vi "Main.vi"(11 "Module Admin":refnum<class "Delacor_lib_QMH_Module Admin.lvclass">) -> ()   [LabVIEW 2024, in "Acquisition.lvlib"]
doc: "This template is based off of the Queued Message Handler design pattern and the Queued Message Handler project template that ships with LabVIEW.\n\nThe main difference is that the queue is private to this module and communication between modules is performed via Broadcast and Request events.\n\nRequest events are wrapped in public API methods and are handled in the Event Handling Loop (EHL) of this VI. Any module can register for Broadcast events sent by this module. The EHL generates messages based on user interface actions.\n\nThe Message Handling Loop (MHL) processes messages generated by the EHL, or by other messages. The messages are string values, so new messages can be added easily to the Message Cases case structure in the MHL. Each message cluster can also provide an optional value for Message Data, which is a variant that can be converted to whatever message-specific data is required.\n_____\nBased on DQMH Project Template 4.0.0.47.\n_____\nBased on DQMH Project Template 7.0.1.1316."
uses:
  Acquisition.lvlib
  <vilib>/Delacor/Delacor QMH/Libraries/Module Admin_class/Delacor_lib_QMH_Module Admin.lvclass
  Module Data--cluster.ctl
  CML Shared/Signal Type--enum.ctl
  CML Shared/Calibration Values--cluster.ctl
  Stop Argument--cluster.ctl
  <vilib>/Delacor/Delacor QMH/Libraries/Message Queue_class/Delacor_lib_QMH_Message Queue.lvclass/Delacor_lib_QMH_Message Queue.ctl
  <vilib>/Delacor/Delacor QMH/Libraries/Module Admin_class/Delacor_lib_QMH_Module Admin.lvclass/Delacor_lib_QMH_Module Admin.ctl
  Start Acquiring Argument--cluster.ctl
  Start Acquiring (Reply Payload)--cluster.ctl
  Stop Acquiring Argument--cluster.ctl
  Settings Editor/Update Application Settings (Reply Payload)--cluster.ctl
  Settings Editor/Settings--cluster.ctl
  <vilib>/Utility/miscctls.llb/LVPointTypeDef.ctl
  <vilib>/Delacor/Delacor QMH/Libraries/Message Queue_class/Delacor_lib_QMH_Enqueue Message (Single).vi
  <vilib>/Delacor/Delacor QMH/Libraries/Module Admin_class/Delacor_lib_QMH_Get External Launch.vi
  <vilib>/Delacor/Delacor QMH/Libraries/Message Queue_class/Delacor_lib_QMH_Message Queue.lvclass
  CML Shared/CML Shared.lvlib
  Settings Editor/Settings Editor.lvlib
  Logger/Logger.lvlib
panel:
  out "Settings":T1
  out "Graph Data":waveform(dbl)[](array[waveform])
  out "error out":errorcluster
  # "This is a headless module. Show its panel to confirm that the Settings are updated correctly and other debugging tasks. Use the Settings Editor to change the settings for this module."
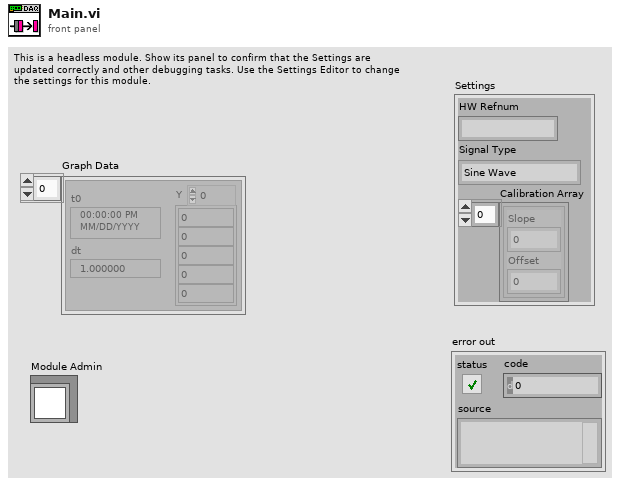
[diagram p1: front panel]
types:
  T1 = typedef "Acquisition.lvlib/Module Data--cluster.ctl" = cluster{"HW Refnum":string, "Signal Type":T2, "Calibration Array":T3[]}
  T2 = typedef "CML Shared.lvlib/Signal Type--enum.ctl" = enum16{"Sine Wave", "Square with Noise"}
  T3 = typedef "CML Shared.lvlib/Calibration Values--cluster.ctl" = cluster{"Slope":dbl, "Offset":dbl}
  T4 = typedef "Settings Editor.lvlib/Broadcast Events--cluster.ctl" = cluster{"Module Did Init":refnum<user-event>, "Status Updated":refnum<user-event>, "Error Reported":refnum<user-event>, "Module Did Stop":refnum<user-event>, "Update Module Execution Status":refnum<user-event>, "Application Settings Updated":refnum<user-event>}
  T5 = typedef "Acquisition.lvlib/Request Events--cluster.ctl" = cluster{"Stop Module":refnum<user-event>, "Show Panel":refnum<user-event>, "Hide Panel":refnum<user-event>, "Get Module Execution Status":refnum<user-event>, "Show Diagram":refnum<user-event>, "Stop Acquiring":refnum<user-event>, "Wakeup Helper Loop":refnum<user-event>, "Change Settings":refnum<user-event>, "Calibrate DAQ":refnum<user-event>, "Start Acquiring":refnum<user-event>}
  T6 = enum32{"invalid lock state", "Not Locked", "Locked (No Password)", "Password-protected"}
  T7 = typedef "Acquisition.lvlib/Stop Argument--cluster.ctl" = cluster{"Origin":string, "Exit via Stop Module Req?":bool, "Wait for Module to stop?":bool}
  T8 = typedef "Acquisition.lvlib/Start Acquiring Argument--cluster.ctl" = cluster{"Wait Notifier":refnum<notifier>, "wait for reply":bool}
  T9 = typedef "Acquisition.lvlib/Stop Acquiring Argument--cluster.ctl" = cluster{"Boolean":bool}
  T10 = typedef "Settings Editor.lvlib/Update Application Settings (Reply Payload)--cluster.ctl" = cluster{"Settings":T11, "error":errorcluster}
  T11 = typedef "Settings Editor.lvlib/Settings--cluster.ctl" = cluster{"Signal Type":T2, "Calibration Array":T3[], "Log File Base Path":path}
  T12 = typedef "LVPointTypeDef.ctl" = cluster{"Horizontal":i16, "Vertical":i16}
  T13 = enum32{"Invalid", "Standard", "Closed", "Hidden", "Minimized", "Maximized"}
  T14 = typedef "Acquisition.lvlib/Start Acquiring (Reply Payload)--cluster.ctl" = cluster{"HW ID":string, "error":errorcluster}
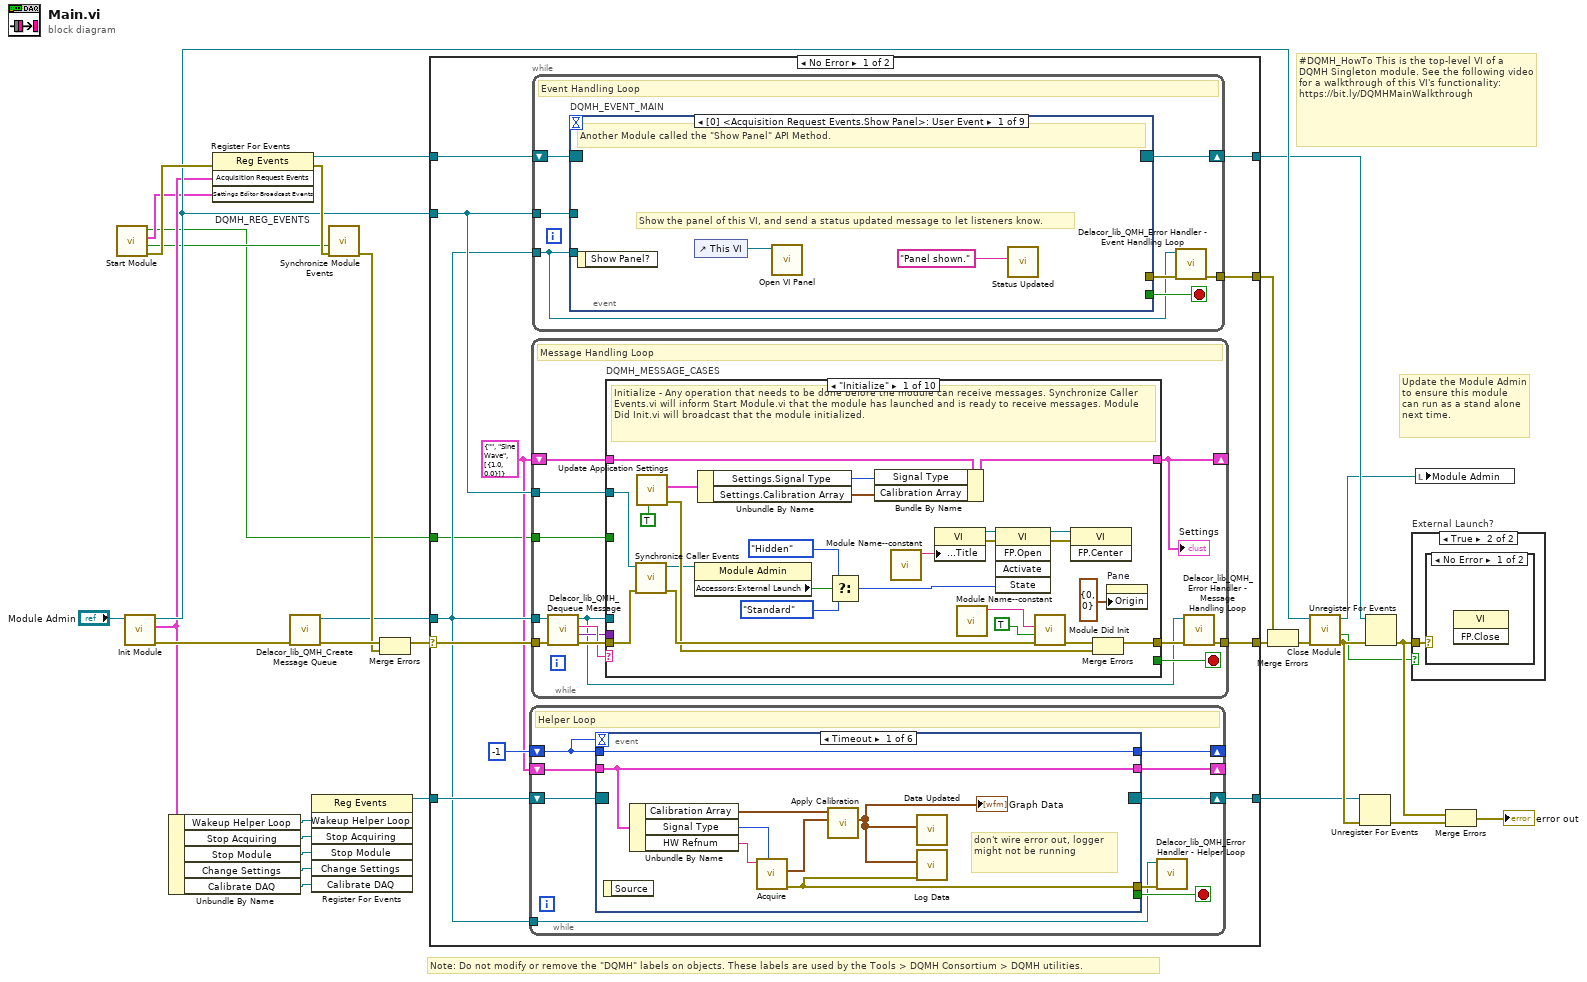
[diagram p0: block diagram]
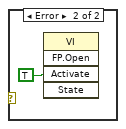
[diagram p3: hidden frame]
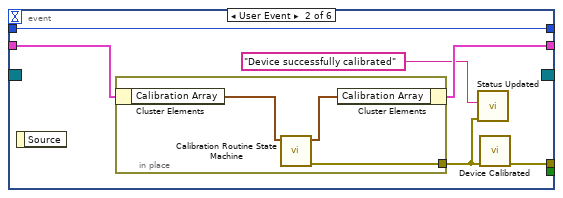
[diagram p4: hidden frame]
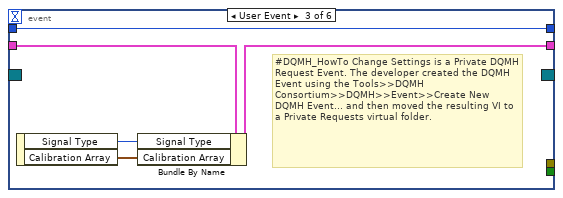
[diagram p5: hidden frame]
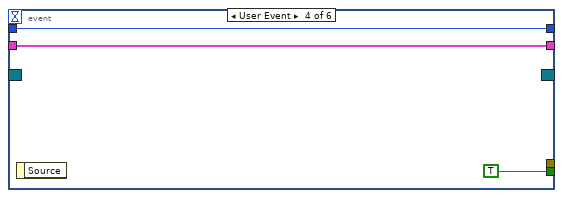
[diagram p6: hidden frame]
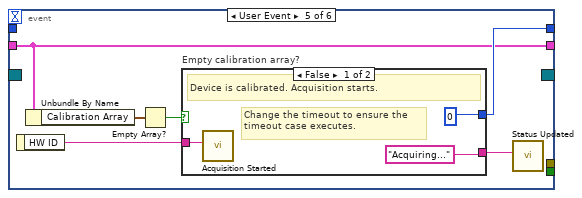
[diagram p7: hidden frame]
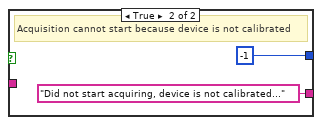
[diagram p8: hidden frame]
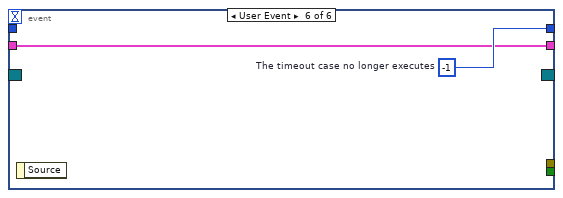
[diagram p9: hidden frame]
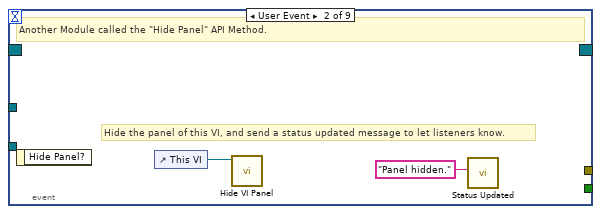
[diagram p10: hidden frame]
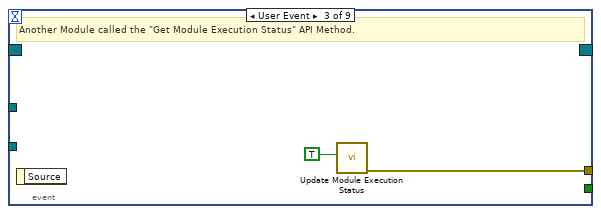
[diagram p11: hidden frame]
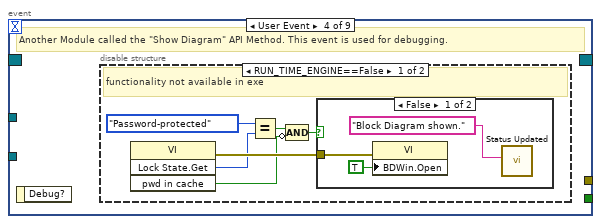
[diagram p12: hidden frame]
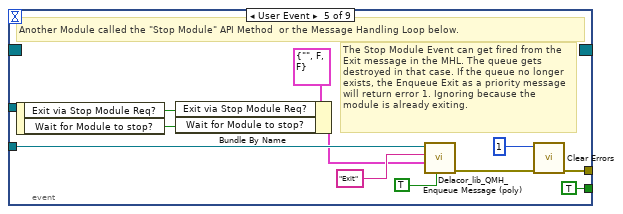
[diagram p15: hidden frame]
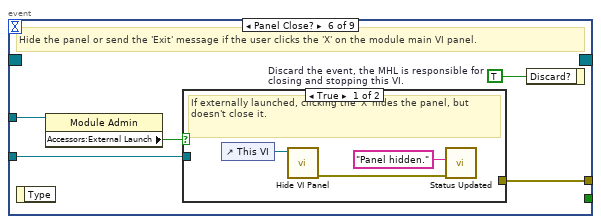
[diagram p16: hidden frame]
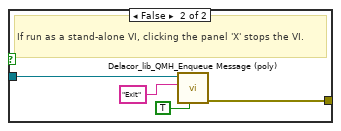
[diagram p17: hidden frame]
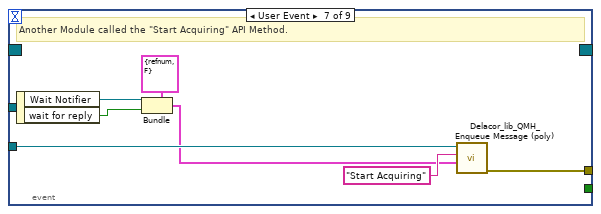
[diagram p18: hidden frame]
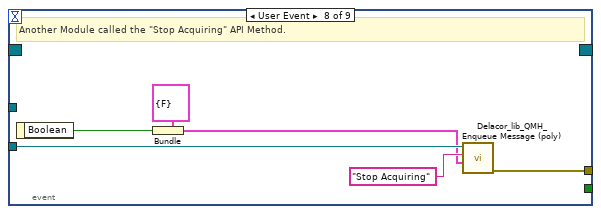
[diagram p19: hidden frame]
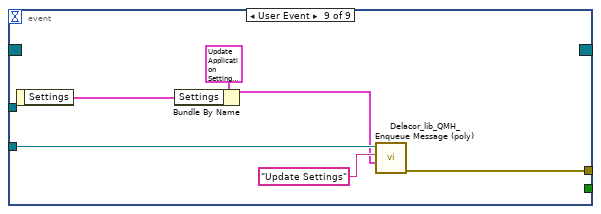
[diagram p20: hidden frame]
diagram:
  # "#DQMH_HowTo This is the top-level VI of a DQMH Singleton module. See the following video for a walkthrough of this VI's functionality: https://bit.ly/DQMHMainWalkthrough"
  # "Note: Do not modify or remove the \"DQMH\" labels on objects. These labels are used by the Tools > DQMH Consortium > DQMH utilities."
  # "Update the Module Admin to ensure this module can run as a stand alone next time."
  n1 = call "Start Module.vi"() -> ("error out"=w24:errorcluster, "Wait for Event Sync?"=w5:bool, "Settings Editor Broadcast Events"=w6:T4, "Module Was Already Running?"=w1:bool)  [unwired: 8 in]
  n2 = call "Init Module.vi"("Singleton Module Admin in"="Module Admin") -> ("error out"=w30:errorcluster, "Acquisition Request Events"=w11:T5, "Singleton Module Admin out"=w18:refnum<class "Delacor_lib_QMH_Module Admin.lvclass">)  [unwired: 8 in]
  n3 = Unbundle By Name(w11) -> ("Wakeup Helper Loop"=w7:refnum<user-event>, "Stop Acquiring"=w10:refnum<user-event>, "Stop Module"=w9:refnum<user-event>, "Change Settings"=w4:refnum<user-event>, "Calibrate DAQ"=w3:refnum<user-event>)
  n4 = register-events "DQMH_REG_EVENTS"(error in=w24, w11, w6) -> (reference out=w16:refnum<event-registration>, error out=w23:errorcluster)  [unwired: 1 in]
  n5 = call <vilib>:"Delacor_lib_QMH_Create Message Queue.vi"("error in"=w30) -> ("error out"=w26:errorcluster, "Message Queue"=w15:refnum<class "Delacor_lib_QMH_Message Queue.lvclass">)  [unwired: 9 in]
  n6 = register-events(w7, w10, w9, w4, w3) -> (reference out=w8:refnum<event-registration>)  [unwired: 2 in, 1 out]
  n7 = call "Synchronize Module Events.vi"("error in"=w23, "Wait for Event Sync?"=w5) -> ("error out"=w22:errorcluster)  [unwired: 9 in]
  n8 = Merge Errors(w26, w22) -> (w25:errorcluster)
  n9 = case shown="No Error" w25 {
    selector: w25 -> [w41 w293]
    tunnel: [w43 w292] -> w31
    tunnel: [w40 w291] -> w17
    tunnel: w16 -> [w39 w291]
    tunnel: w15 -> [w35 w284]
    tunnel: [w42 _] -> w29
    tunnel: w18 -> [w38 w287]
    tunnel: w8 -> [w36 w286]
    tunnel: [w33 w286] -> w2
    tunnel: w1 -> [w32 w285]
    frame No Error {
      w34 = T1 {"HW Refnum"="", "Signal Type"=enum."Sine Wave", "Calibration Array"=[{"Slope"=1.0, "Offset"=0.0}]} ("Data Cluster")
      n10 = while {
        shift-right: [w51] -> _
        shift-left: -1 -> [w50]
        tunnel: w35 -> [w44]
        shift-right: [w47] -> _
        shift-left: w34 -> [w46]
        shift-right: [w45] -> w33
        shift-left: w36 -> [w49]
        stop <- w48 stop-if-true
        # "Helper Loop"
        n11 = event shown="[0] Timeout" {
          selector: w49 -> [_ _ _ _ _ _]
          dyn-events: [_ _ _ _ _ _] -> w45
          timeout: w50 -> [_ _ _ _ _ _]
          tunnel: [w59 w64 w74 w77 w82 w90] -> w51
          tunnel: w50 -> [w59 w64 w74 w77 _ _]
          tunnel: [_ _ _ TRUE _ _] -> w48
          tunnel: [w60 w66 _ _ _ _] -> w52
          tunnel: [w56 w62 w72 w75 w79 w89] -> w47
          tunnel: w46 -> [w56 w63 w73 w75 w79 w89]
          event Timeout {
            # "don't wire error out, logger might not be running"
            n12 = event-data() -> ()  [unwired: 1 in, 1 out]
            n13 = Unbundle By Name(w56) -> ("Calibration Array"=w54:T3[], "Signal Type"=w58:T2, "HW Refnum"=w57:string)
            n14 = call "Acquire.vi"("Signal Type"=w58, "HW ID in"=w57) -> ("error out"=w60:errorcluster, "Graph Data"=w55:waveform(dbl)[])  [unwired: 7 in, 1 out]
            n15 = call "Apply Calibration.vi"("Graph Data"=w55, "Calibration Array"=w54) -> ("Calibrated Data"=w53:waveform(dbl)[])  [unwired: 9 in]
            "Graph Data" <- w53
            n16 = call "Data Updated.vi"("Graph Data"=w53) -> ()  [unwired: 10 in, 1 out]
            n17 = call "Log Data.vi"("error in"=w60, "Waveforms"=w53) -> ()  [unwired: 9 in, 1 out]
          }
          event User Event {
            n18 = event-data() -> ()  [unwired: 1 in, 1 out]
            n19 = in-place {
              in-place-border: [w69] -> w65
              n20 = in-place-cluster #1(w63) -> ("Calibration Array"=w68:T3[])
              n21 = call "Calibration Routine State Machine.vi"("Calibration Array in"=w68) -> ("error out"=w69:errorcluster, "Calibration Array out"=w67:T3[])  [unwired: 9 in]
              n22 = in-place-cluster #1("Calibration Array"=w67) -> (w62:T1)
            }
            n23 = call "Status Updated.vi"("error in"=w65, "Status"="Device successfully calibrated") -> ()  [unwired: 9 in, 1 out]
            n24 = call "Device Calibrated.vi"("error in"=w65) -> ("error out"=w66:errorcluster)  [unwired: 10 in]
          }
          event User Event {
            # "#DQMH_HowTo Change Settings is a Private DQMH Request Event. The developer created the DQMH Event using the Tools>>DQMH Consortium>>DQMH>>Event>>Create New DQMH Event... and then moved the resulting VI to a Private Requests virtual folder."
            n25 = event-data() -> ("Signal Type"=w71:T2, "Calibration Array"=w70:T3[])  [unwired: 1 in]
            n26 = Bundle By Name(cluster=w73, "Signal Type"=w71, "Calibration Array"=w70) -> (w72:T1)
          }
          event User Event {
            n27 = event-data() -> ()  [unwired: 1 in, 1 out]
          }
          event User Event {
            n28 = event-data() -> ("HW ID"=w80:string)  [unwired: 1 in]
            n29 = Unbundle By Name(w79) -> ("Calibration Array"=w78:T3[])
            n30 = Empty Array?(array=w78) -> (empty?=w83:bool)
            n31 = case "Empty calibration array?" shown="False" w83 {
              tunnel: ["Acquiring..." ("Status") "Did not start acquiring, device is not calibrated..." ("Status")] -> w81
              tunnel: [0 -1] -> w82
              tunnel: w80 -> [w86 _]
              frame False {
                # "Change the timeout to ensure the timeout case executes."
                # "Device is calibrated. Acquisition starts."
                n32 = call "Acquisition Started.vi"("HW ID"=w86) -> ()  [unwired: 10 in, 1 out]
              }
              frame True {
                # "Acquisition cannot start because device is not calibrated"
              }
            }
            n33 = call "Status Updated.vi"("Status"=w81) -> ()  [unwired: 10 in, 1 out]
          }
          event User Event {
            w90 = -1  # The timeout case no longer executes
            n34 = event-data() -> ()  [unwired: 1 in, 1 out]
          }
        }
        n35 = call-dynamic "Delacor_lib_QMH_Error Handler - Helper Loop.vi"("error in"=w52, "Message Queue in"=w44) -> ()  [unwired: 8 in, 2 out]
      }
      n36 = while {
        tunnel: w35 -> [w158]
        shift-right: [w162] -> _
        shift-left: w34 -> [w163]
        tunnel: w41 -> [w166]
        tunnel: [w164] -> w43
        tunnel: w38 -> [w156]
        tunnel: w32 -> [w155]
        stop <- w161 stop-if-true
        # "Message Handling Loop"
        n37 = call-dynamic "Delacor_lib_QMH_Dequeue Message.vi"("error in"=w166, "Message Queue in"=w158) -> ("error out"=w165:errorcluster, "Message Data"=w159:variant, "Message"=w160:string, "Message Queue out"=w157:refnum<class "Delacor_lib_QMH_Message Queue.lvclass">)  [unwired: 6 in]
        n38 = case "DQMH_MESSAGE_CASES" shown="\"Initialize\"" w160 {
          selector: w160 -> [_ _ _ _ _ _ _ _ _ w279]
          tunnel: w157 -> [_ _ _ _ _ _ _ w240 w264 _]
          tunnel: w165 -> [w190 w194 w207 w221 w231 w234 w236 w247 w271 w282]
          tunnel: [w187 w194 w205 w219 w229 w233 w236 w243 w265 w283] -> w167
          tunnel: w163 -> [w177 w193 w195 w216 w227 w232 w235 w242 w256 w280]
          tunnel: [w172 w193 w203 w216 w227 w232 w235 w242 w256 w280] -> w162
          tunnel: [_ _ _ _ _ _ _ _ w263 _] -> w161
          tunnel: w159 -> [_ _ w202 w218 w228 _ _ w241 w262 _]
          tunnel: w156 -> [w178 _ _ _ _ _ _ w239 w257 _]
          tunnel: w155 -> [_ _ _ _ _ _ _ _ w254 _]
          frame "Initialize" {
            # "Initialize - Any operation that needs to be done before the module can receive messages. Synchronize Caller Events.vi will inform Start Module.vi that the module has launched and is ready to receive messages. Module Did Init.vi will broadcast that the module initialized."
            n39 = call "Synchronize Caller Events.vi"("error in"=w190, "Singleton Module Admin in"=w178) -> ("error out"=w189:errorcluster, "Singleton Module Admin out"=w174:refnum<class "Delacor_lib_QMH_Module Admin.lvclass">)  [unwired: 8 in]
            n40 = call "Update Application Settings.vi"("wait for reply (T)"=TRUE) -> ("error out"=w186:errorcluster, "Reply Payload"=w171:T10)  [unwired: 8 in, 1 out]
            n41 = property on="Property Node" class="Module Admin"(reference=w174) -> ("Accessors:External Launch"=w182:bool)  [unwired: 1 in, 2 out]
            n42 = Unbundle By Name(w171) -> ("Settings.Signal Type"=w170:T2, "Settings.Calibration Array"=w169:T3[])
            n43 = Select(t=T13."Hidden" ("State"), s=w182, f=T13."Standard" ("State")) -> (s? t:f=w179:T13)
            n44 = Bundle By Name(cluster=w177, "Signal Type"=w170, "Calibration Array"=w169) -> (w172:T1)
            n45 = call "Module Name--constant.vi"() -> ("Module Name"=w185:string)  [unwired: 11 in]
            n46 = property on="Property Node" class="VI"("Front Panel.Title"=w185) -> (reference out=w184:refnum<vi>, error out=w192:errorcluster)  [unwired: 2 in]
            n47 = call "Module Name--constant.vi"() -> ("Module Name"=w175:string)  [unwired: 11 in]
            n48 = invoke on="Invoke Node" class="VI" method="FP.Open"(reference=w184, error in=w192, "State"=w179) -> (reference out=w183:refnum<vi>, error out=w191:errorcluster)  [unwired: 2 in, 3 out]
            n49 = call "Module Did Init.vi"("error in"=w189, "Initialized?"=TRUE, "Origin"=w175) -> ("error out"=w188:errorcluster)  [unwired: 8 in]
            n50 = invoke on="Invoke Node" class="VI" method="FP.Center"(reference=w183, error in=w191) -> ()  [unwired: 1 in, 3 out]
            n51 = Merge Errors(w188, w186) -> (w187:errorcluster)
            n52 = property on="Pane" class="Pane"("Origin"=T12 {"Horizontal"=0, "Vertical"=0}) -> ()  [unwired: 2 in, 2 out]
          }
          frame "---Module Specific---" {
            # "Separator -- The following cases handle messages specific to this Module."
          }
          frame "Start Acquiring" {
            # "Requests Acquisition Module to start acquiring."
            n53 = Variant To Data(error in=w207, type=T8 {"Wait Notifier"=refnum, "wait for reply"=FALSE} ("Start Acquisition Argument"), Variant=w202) -> (data=w200:T8, error out=w204:errorcluster)
            n54 = in-place {
              in-place-border: [w213] -> w206
              in-place-border: w204 -> [w212]
              in-place-border: [w208] -> w196
              n55 = in-place-cluster #2(w195) -> ("HW Refnum"=w209:string)
              n56 = call "Initialize Hardware References.vi"("error in"=w212, "HW Refnum in"=w209) -> ("error out"=w211:errorcluster, "HW Refnum out"=w210:string)  [unwired: 8 in]
              n57 = call "Configure Hardware.vi"("error in"=w211, "HW Refnum in"=w210) -> ("error out"=w213:errorcluster, "HW Refnum out"=w208:string)  [unwired: 8 in]
              n58 = in-place-cluster #2("HW Refnum"=w208) -> (w203:T1)
            }
            n59 = Unbundle By Name(w200) -> ("Wait Notifier"=w199:refnum<notifier>)
            n60 = call "Wakeup Helper Loop.vi"("error in"=w206, "HW ID"=w196) -> ("error out"=w205:errorcluster)  [unwired: 9 in]
            n61 = Bundle By Name(cluster=T14 {"HW ID"="", "error"={"status"=FALSE, "code"=0, "source"=""}} ("Start Acquisition (Reply Payload)"), "HW ID"=w196, "error"=w206) -> (w198:T14)
            n62 = Send Notification(notification=w198, notifier=w199) -> ()  [unwired: 1 in, 2 out]
          }
          frame "Stop Acquiring" {
            # "Requests the Acquisition Module to stop acquiring"
            n63 = Variant To Data(error in=w221, type=T9 {"Boolean"=FALSE} ("Stop Acquiring Argument"), Variant=w218) -> (error out=w220:errorcluster)  [unwired: 1 out]
            n64 = Unbundle By Name(w216) -> ("HW Refnum"=w215:string)
            n65 = call "Stop Acquisition.vi"("error in"=w220, "HW Refnum"=w215) -> ("error out"=w219:errorcluster)  [unwired: 9 in]
            n66 = call "Acquisition Stopped.vi"("error in"=w219) -> ()  [unwired: 10 in, 1 out]
            n67 = call "Status Updated.vi"("error in"=w219, "Status"="Acquisition Stopped") -> ()  [unwired: 9 in, 1 out]
          }
          frame "Update Settings" {
            # "Send the Change Settings event to the helper loop."
            # "The Settings Editor broadcasted that the settings have changed."
            n68 = Variant To Data(error in=w231, type=T10 {"Settings"={"Signal Type"=enum."Sine Wave", "Calibration Array"=[], "Log File Base Path"=path ""}, "error"={"status"=FALSE, "code"=0, "source"=""}} ("Settings Updated Argument"), Variant=w228) -> (data=w225:T10, error out=w230:errorcluster)
            n69 = Unbundle By Name(w225) -> ("Settings.Signal Type"=w224:T2, "Settings.Calibration Array"=w222:T3[])
            n70 = call "Change Settings.vi"("error in"=w230, "Calibration Array"=w222, "Signal Type"=w224) -> ("error out"=w229:errorcluster)  [unwired: 8 in]
            n71 = call "Status Updated.vi"("error in"=w229, "Status"="Settings Updated") -> ()  [unwired: 9 in, 1 out]
          }
          frame "---Copy This Frame---" {
            # "Duplicate this frame when creating new messages.  Change this comment in the duplicated frame to describe this message."
            n72 = Merge Errors(w234) -> (w233:errorcluster)
          }
          frame "---Exit and Error Handling---" {
            # "Separator - The following cases handle errors and exit messages."
          }
          frame "Error" {
            # "Error - Check the error message data and respond accordingly. This message is sent by the \"Error Handler\" VIs at the end of each loop in this application."
            n73 = property on="Property Node" class="Module Admin"(reference=w239) -> ("Accessors:External Launch"=w238:bool)  [unwired: 1 in, 2 out]
            n74 = Variant To Data(error in=w247, type=errorcluster {"status"=FALSE, "code"=0, "source"=""} ("error constant"), Variant=w241) -> (data=w237:errorcluster, error out=w245:errorcluster)
            n75 = local write "error out"(w237) -> ()
            n76 = call "Error Reported.vi"("Error"=w237) -> ()  [unwired: 10 in, 1 out]
            n77 = case shown="False" w238 {
              tunnel: [w252 _] -> w244
              tunnel: w240 -> [w250 _]
              tunnel: w237 -> [w251 _]
              frame False {
                n78 = disable-structure shown="Default" {
                  disable-tunnel: w251 -> [w253 _]
                  frame condition #0 (active) {
                    # "If the module is running standalone, then pop up an error dialog and call the \"Exit\" message."
                    n79 = call <vilib>:"Simple Error Handler.vi"("error in (no error)"=w253) -> ()  [unwired: 4 in, 5 out]
                  }
                  frame condition #1 {
                    # "To prevent the Simple Error Handler VI from being loaded (e.g. when deploying to a Real-Time target), add the Conditional Disable Symbol \"DQMH_Disable_SEH\" to your project and set it to TRUE."
                  }
                }
                n80 = call-poly <vilib>:"Delacor_lib_QMH_Enqueue Message (poly).vi"("Priority Message? (F)"=TRUE, "Message"="Exit", "Message Queue in"=w250) -> ("error out"=w252:errorcluster)  [unwired: 7 in, 1 out]
              }
              frame True {
                # "If the module was launched externally, calling the Error Reported broadcast VI is the only action performed by the \"Error\" message. The module's caller can then process the error appropriately."
              }
            }
            n81 = Merge Errors(w245, w244) -> (w243:errorcluster)
          }
          frame "Exit" {
            w263 = TRUE  # Stop the VI
            # "Release the message queue reference"
            # "Exit - Exit the application."
            n82 = Variant To Data(error in=w271, type=T7 {"Origin"="", "Exit via Stop Module Req?"=FALSE, "Wait for Module to stop?"=FALSE} ("Stop Argument"), Variant=w262) -> (data=w259:T7, error out=w268:errorcluster)
            n83 = call <vilib>:"Clear Errors.vi"("error in (no error)"=w268, "specific error code to clear (0: all)"=91 ("91: not all Exit messages will have an argument")) -> ("error out"=w270:errorcluster)  [unwired: 4 in, 1 out]
            n84 = Unbundle By Name(w256) -> ("HW Refnum"=w255:string)
            n85 = control-ref of="This VI"() -> (w258:refnum<vi>)
            n86 = call "Handle Exit.vi"("Stop Argument"=w259, "Admin in"=w257, "VI reference"=w258) -> ("error out"=w267:errorcluster)  [unwired: 7 in, 1 out]
            n87 = call "Close Hardware References.vi"("HW Refnum in"=w255) -> ("error out"=w266:errorcluster)  [unwired: 9 in, 1 out]
            n88 = call-dynamic "Delacor_lib_QMH_Release Message Queue.vi"("error in"=w270, "Message Queue"=w264) -> ("error out"=w269:errorcluster)  [unwired: 9 in]
            n89 = case "Settings Editor was\nalready running?" shown="False" w254 {
              frame False {
                n90 = call "Module Name--constant.vi"() -> ("Module Name"=w273:string)  [unwired: 11 in]
                n91 = call "Stop Module.vi"("Wait for Module to Stop? (F)"=TRUE, "Origin"=w273) -> ()  [unwired: 9 in, 1 out]
              }
              frame True {
                # "Another Module stops the Settings Editor"
              }
            }
            n92 = Merge Errors(w269, w267, w266) -> (w265:errorcluster)
            n93 = call "Error Reported.vi"("Error"=w265) -> ()  [unwired: 10 in, 1 out]
          }
          frame Default {
            # "'Default' case only runs if there is a message that isn't defined in any of the other cases.  Output a programming error."
            n94 = call "Module Name--constant.vi"() -> ("Module Name"=w278:string)  [unwired: 11 in]
            n95 = Format Into String(format string="The invalid message string \"%s\" was received in the Message Handling Loop for module \"%s\".", w279, w278) -> (resulting string=w276:string)  [unwired: 2 in, 1 out]
            n96 = call <vilib>:"Error Cluster From Error Code.vi"("show call chain? (False)"=TRUE, "error message (\"\")"=w276, "error code (0)"=1) -> ("error out"=w281:errorcluster)  [unwired: 6 in]
            n97 = Merge Errors(w282, w281) -> (w283:errorcluster)
          }
        }
        "Settings" <- w162
        n98 = call-dynamic "Delacor_lib_QMH_Error Handler - Message Handling Loop.vi"("error in"=w167, "Message Queue in"=w157) -> ("dup error in"=w164:errorcluster)  [unwired: 8 in, 1 out]
      }
      n99 = while {
        tunnel: w35 -> [w91]
        shift-right: [w94] -> w40
        shift-left: w39 -> [w95]
        tunnel: [w96] -> w42
        tunnel: w38 -> [w92]
        stop <- w93 stop-if-true
        # "Event Handling Loop"
        n100 = event "DQMH_EVENT_MAIN" shown="[0] <Acquisition Request Events.Show Panel>: User Event" {
          selector: w95 -> [_ _ _ _ _ _ _ _ _]
          dyn-events: [_ _ _ _ _ _ _ _ _] -> w94
          timeout: _ -> [_ _ _ _ _ _ _ _ _]
          tunnel: [_ _ _ _ TRUE ("Discard?") _ _ _ _] -> w93
          tunnel: w91 -> [_ _ _ _ w119 w126 w141 w147 w152]
          tunnel: [_ _ w103 _ w122 w128 w142 w148 w154] -> w97
          tunnel: w92 -> [_ _ _ _ _ w125 _ _ _]
          event User Event {
            # "Show the panel of this VI, and send a status updated message to let listeners know."
            # "Another Module called the \"Show Panel\" API Method."
            n101 = event-data() -> ()  [unwired: 1 in, 1 out]
            n102 = control-ref of="This VI"() -> (w99:refnum<vi>)
            n103 = call "Open VI Panel.vi"("VI"=w99) -> ()  [unwired: 10 in, 1 out]
            n104 = call "Status Updated.vi"("Status"="Panel shown." ("format string")) -> ()  [unwired: 10 in, 1 out]
          }
          event User Event {
            # "Hide the panel of this VI, and send a status updated message to let listeners know."
            # "Another Module called the \"Hide Panel\" API Method."
            n105 = event-data() -> ()  [unwired: 1 in, 1 out]
            n106 = control-ref of="This VI"() -> (w101:refnum<vi>)
            n107 = call "Hide VI Panel.vi"("VI"=w101) -> ()  [unwired: 10 in, 1 out]
            n108 = call "Status Updated.vi"("Status"="Panel hidden." ("format string")) -> ()  [unwired: 10 in, 1 out]
          }
          event User Event {
            # "Another Module called the \"Get Module Execution Status\" API Method."
            n109 = event-data() -> ()  [unwired: 1 in, 1 out]
            n110 = call "Update Module Execution Status.vi"("Running?"=TRUE) -> ("error out"=w103:errorcluster)  [unwired: 10 in]
          }
          event User Event {
            # "Another Module called the \"Show Diagram\" API Method. This event is used for debugging."
            n111 = event-data() -> ()  [unwired: 1 in, 1 out]
            n112 = disable-structure shown="RUN_TIME_ENGINE==False" {
              frame condition #0 (active) {
                # "functionality not available in exe"
                n113 = invoke on="Invoke Node" class="VI" method="Lock State.Get"() -> (error out=w109:errorcluster, "Get Lock State"=w108:T6, "pwd in cache"=w105:bool)  [unwired: 4 in, 1 out]
                n114 = Equal?(x=T6."Password-protected", y=w108) -> (x = y?=w106:bool)
                n115 = Compound Arithmetic op=AND(w106, invert w105) -> (w104:bool)
                n116 = case shown="False" w104 {
                  tunnel: w109 -> [w112 _]
                  frame False {
                    n117 = property on="Property Node" class="VI"(error in=w112, "BDWin.Open"=TRUE ("Block Diagram Window:Open")) -> ()  [unwired: 1 in, 2 out]
                    n118 = call "Status Updated.vi"("Status"="Block Diagram shown." ("format string")) -> ()  [unwired: 10 in, 1 out]
                  }
                  frame True {
                    # "Password-protected VI, and the password is not in the cache. Do not show the diagram."
                  }
                }
              }
              frame condition #1 {
              }
            }
          }
          event User Event {
            # "The Stop Module Event can get fired from the Exit message in the MHL. The queue gets destroyed in that case. If the queue no longer exists, the Enqueue Exit as a priority message will return error 1. Ignoring because the module is already exiting."
            # "Another Module called the \"Stop Module\" API Method  or the Message Handling Loop below."
            n119 = event-data() -> ("Exit via Stop Module Req?"=w115:bool, "Wait for Module to stop?"=w114:bool)  [unwired: 1 in]
            n120 = Bundle By Name(cluster=T7 {"Origin"="", "Exit via Stop Module Req?"=FALSE, "Wait for Module to stop?"=FALSE} ("Stop Argument"), "Exit via Stop Module Req?"=w115, "Wait for Module to stop?"=w114) -> (w113:T7)
            n121 = call-poly <vilib>:"Delacor_lib_QMH_Enqueue Message (poly).vi"("Priority Message? (F)"=TRUE, "Message Data"=w113, "Message"="Exit", "Message Queue in"=w119) -> ("error out"=w123:errorcluster)  [unwired: 6 in, 1 out]
            n122 = call <vilib>:"Clear Errors.vi"("error in (no error)"=w123, "specific error code to clear (0: all)"=1) -> ("error out"=w122:errorcluster)  [unwired: 4 in, 1 out]
          }
          event Panel Close? {
            w127 = TRUE  # Discard the event, the MHL is responsible for closing and stopping this VI.
            # "Hide the panel or send the 'Exit' message if the user clicks the 'X' on the module main VI panel."
            n123 = event-data() -> ()  [unwired: 1 in, 1 out]
            n124 = property on="Property Node" class="Module Admin"(reference=w125) -> ("Accessors:External Launch"=w124:bool)  [unwired: 1 in, 2 out]
            n125 = case shown="True" w124 {
              tunnel: w126 -> [_ w134]
              tunnel: [_ w135] -> w128
              frame True {
                # "If externally launched, clicking the 'X' hides the panel, but doesn't close it."
                n126 = control-ref of="This VI"() -> (w131:refnum<vi>)
                n127 = call "Hide VI Panel.vi"("VI"=w131) -> ("error out"=w129:errorcluster)  [unwired: 10 in]
                n128 = call "Status Updated.vi"("error in"=w129, "Status"="Panel hidden." ("format string")) -> ()  [unwired: 9 in, 1 out]
              }
              frame False {
                # "If run as a stand-alone VI, clicking the panel 'X' stops the VI."
                n129 = call-poly <vilib>:"Delacor_lib_QMH_Enqueue Message (poly).vi"("Priority Message? (F)"=TRUE, "Message"="Exit", "Message Queue in"=w134) -> ("error out"=w135:errorcluster)  [unwired: 7 in, 1 out]
              }
            }
            n130 = event-data ("Event Filter Node")("Discard?"=w127) -> ()  [unwired: 1 in, 1 out]
          }
          event User Event {
            # "Another Module called the \"Start Acquiring\" API Method."
            n131 = event-data() -> ("Wait Notifier"=w137:refnum<notifier>, "wait for reply"=w136:bool)  [unwired: 1 in]
            n132 = Bundle(cluster=T8 {"Wait Notifier"=refnum, "wait for reply"=FALSE} ("Start Acquisition Argument"), "Wait Notifier"=w137, "wait for reply"=w136) -> (w138:T8)
            n133 = call-poly <vilib>:"Delacor_lib_QMH_Enqueue Message (poly).vi"("Message Data"=w138, "Message"="Start Acquiring", "Message Queue in"=w141) -> ("error out"=w142:errorcluster)  [unwired: 7 in, 1 out]
          }
          event User Event {
            # "Another Module called the \"Stop Acquiring\" API Method."
            n134 = event-data() -> ("Boolean"=w143:bool)  [unwired: 1 in]
            n135 = Bundle(cluster=T9 {"Boolean"=FALSE} ("Stop Acquiring Argument"), "Boolean"=w143) -> (w144:T9)
            n136 = call-poly <vilib>:"Delacor_lib_QMH_Enqueue Message (poly).vi"("Message Data"=w144, "Message"="Stop Acquiring", "Message Queue in"=w147) -> ("error out"=w148:errorcluster)  [unwired: 7 in, 1 out]
          }
          event User Event {
            n137 = event-data() -> ("Settings"=w149:T11)  [unwired: 1 in]
            n138 = Bundle By Name(cluster=T10 {"Settings"={"Signal Type"=enum."Sine Wave", "Calibration Array"=[], "Log File Base Path"=path ""}, "error"={"status"=FALSE, "code"=0, "source"=""}} ("Settings Updated Argument"), "Settings"=w149) -> (w151:T10)
            n139 = call-poly <vilib>:"Delacor_lib_QMH_Enqueue Message (poly).vi"("Message Data"=w151, "Message"="Update Settings", "Message Queue in"=w152) -> ("error out"=w154:errorcluster)  [unwired: 7 in, 1 out]
          }
        }
        n140 = call-dynamic "Delacor_lib_QMH_Error Handler - Event Handling Loop.vi"("error in"=w97, "Message Queue in"=w91) -> ("dup error in"=w96:errorcluster)  [unwired: 8 in, 1 out]
      }
    }
    frame Error {
      # "Synchronize Caller Events.vi will inform Start Module.vi that the module has launched and will let the code calling Start Module.vi register for broadcasts and would permit the caller receive the broadcast that an error occurred at launch time."
      n141 = call "Synchronize Caller Events.vi"("Singleton Module Admin in"=w287) -> ("error out"=w294:errorcluster)  [unwired: 9 in, 1 out]
      n142 = call-dynamic "Delacor_lib_QMH_Release Message Queue.vi"("error in"=w293, "Message Queue"=w284) -> ("error out"=w292:errorcluster)  [unwired: 9 in]
      n143 = call "Module Name--constant.vi"() -> ("Module Name"=w290:string)  [unwired: 11 in]
      n144 = case "Settings Editor was\nalready running?" shown="False" w285 {
        frame False {
          n145 = call "Module Name--constant.vi"() -> ("Module Name"=w297:string)  [unwired: 11 in]
          n146 = call "Stop Module.vi"("Wait for Module to Stop? (F)"=TRUE, "Origin"=w297) -> ()  [unwired: 9 in, 1 out]
        }
        frame True {
          # "Another Module is\nin charge of stopping Settings Editor"
        }
      }
      n147 = Format Into String(format string="An error occurred during initialization. %s is no longer running.", w290) -> (resulting string=w288:string)  [unwired: 2 in, 1 out]
      n148 = Merge Errors(w292, w294) -> (w295:errorcluster)
      n149 = call "Error Reported.vi"("Additional Information"=w288, "Error"=w295) -> ()  [unwired: 9 in, 1 out]
    }
  }
  n150 = Merge Errors(w29, w31) -> (w28:errorcluster)
  n151 = call "Close Module.vi"("error in"=w28, "Module Admin in"=w18) -> ("error out"=w21:errorcluster, "External Launch"=w12:bool, "Module Admin out"=w13:refnum<class "Delacor_lib_QMH_Module Admin.lvclass">)  [unwired: 7 in]
  n152 = Unregister For Events(event registration refnum=w2, error in=w21) -> (error out=w19:errorcluster)
  n153 = Unregister For Events(event registration refnum=w17, error in=w21) -> (error out=w27:errorcluster)
  n154 = case "External Launch?" shown="True" w12 {
    tunnel: w27 -> [_ w298]
    frame False {
    }
    frame True {
      n155 = case shown="No Error" w298 {
        frame No Error {
          n156 = invoke on="Invoke Node" class="VI" method="FP.Close"() -> ()  [unwired: 3 in, 3 out]
        }
        frame Error {
          n157 = invoke on="Invoke Node" class="VI" method="FP.Open"("Activate"=TRUE ("Activate?")) -> ()  [unwired: 4 in, 5 out]
        }
      }
    }
  }
  n158 = local write "Module Admin"(w13) -> ()
  n159 = Merge Errors(w27, w19) -> (→"error out":errorcluster)
